vi "Get Path Regex.vi"(8 "error in (no error)":errorcluster, 11 "Scores in":refnum<class "Leaderboard.lvclass">) -> (0 "error out":errorcluster, 2 "Path Regex":string, 3 "Scores out":refnum<class "Leaderboard.lvclass">)   [LabVIEW 2020, in "Summer of LabVIEW.lvlib" / "Leaderboard.lvclass"]
uses:
  Leaderboard.lvclass
  Leaderboard.lvclass/Leaderboard.ctl
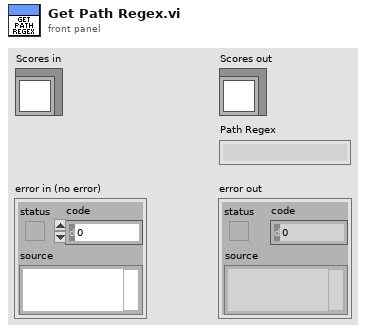
[diagram p1: front panel]
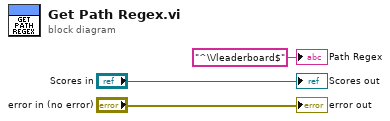
[diagram p0: block diagram]
diagram:
  "error out" <- "error in (no error)"
  "Scores out" <- "Scores in"
  "Path Regex" <- "^\\/leaderboard$" ("Path Regex")
